vi "Read Absolute Max.vi"(8 "error in (no error)":errorcluster, 11 "PowerSupply in":refnum<class "PowerSupply.lvclass">) -> (0 "error out":errorcluster, 3 "PowerSupply out":refnum<class "PowerSupply.lvclass">)   [LabVIEW 2019, in "PowerSupply.lvlib" / "PowerSupply.lvclass"]
uses:
  PowerSupply.lvclass
  PowerSupply.lvclass/PowerSupply.ctl
  Accessors/Read/Read Configuration.vi
  Desktop/Built/Configuration.lvlibp/Configuration.lvclass
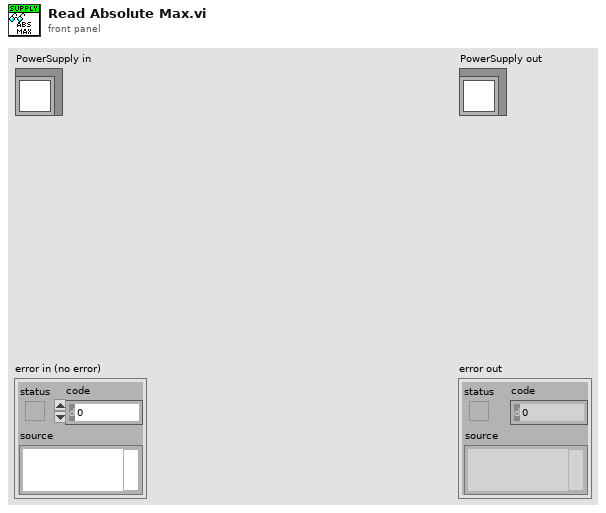
[diagram p1: front panel]
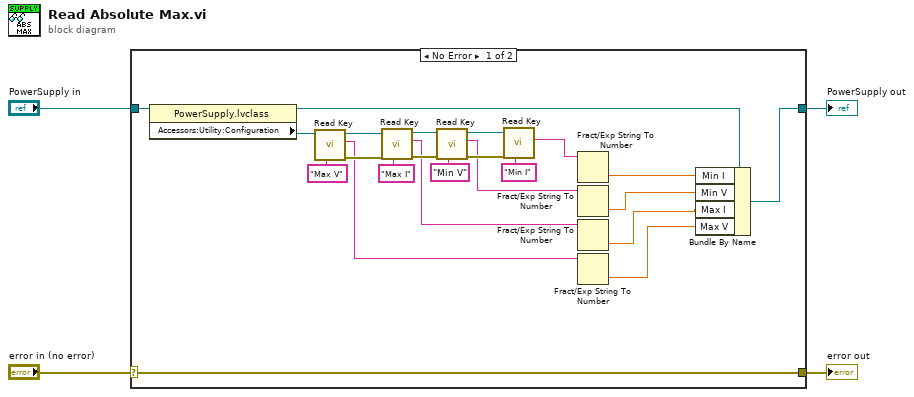
[diagram p0: block diagram]
diagram:
  n1 = case shown="No Error" "error in (no error)" {
    selector: "error in (no error)" -> [w26 w29]
    tunnel: [w26 w29] -> w3
    tunnel: [w13 w28] -> w1
    tunnel: "PowerSupply in" -> [w27 w28]
    frame No Error {
      n2 = property class="PowerSupply.lvclass"(reference=w27) -> (reference out=w25:refnum<class "PowerSupply.lvclass">, "Accessors:Utility:Configuration"=w24:refnum<class "Configuration.lvclass">)  [unwired: 1 in, 1 out]
      n3 = call "Read Key.vi"("Key Name"="Max V", "Configuration in"=w24) -> ("error out"=w22:errorcluster, "Key Value"=w8:string, "Configuration out"=w21:refnum<class "Configuration.lvclass">)  [unwired: 7 in]
      n4 = call "Read Key.vi"("Key Name"="Max I", "error in (no error)"=w22, "Configuration in"=w21) -> ("error out"=w17:errorcluster, "Key Value"=w9:string, "Configuration out"=w16:refnum<class "Configuration.lvclass">)  [unwired: 6 in]
      n5 = call "Read Key.vi"("Key Name"="Min V", "error in (no error)"=w17, "Configuration in"=w16) -> ("error out"=w18:errorcluster, "Key Value"=w10:string, "Configuration out"=w15:refnum<class "Configuration.lvclass">)  [unwired: 6 in]
      n6 = call "Read Key.vi"("Key Name"="Min I", "error in (no error)"=w18, "Configuration in"=w15) -> ("Key Value"=w11:string)  [unwired: 6 in, 2 out]
      n7 = Fract/Exp String To Number(string=w11) -> (number=w12:dbl)  [unwired: 3 in, 1 out]
      n8 = Fract/Exp String To Number(string=w10) -> (number=w7:dbl)  [unwired: 3 in, 1 out]
      n9 = Fract/Exp String To Number(string=w9) -> (number=w6:dbl)  [unwired: 3 in, 1 out]
      n10 = Fract/Exp String To Number(string=w8) -> (number=w5:dbl)  [unwired: 3 in, 1 out]
      n11 = Bundle By Name(cluster=w25, "Min I"=w12, "Min V"=w7, "Max I"=w6, "Max V"=w5) -> (w13:refnum<class "PowerSupply.lvclass">)
    }
    frame Error {
    }
  }
  "error out" <- w3
  "PowerSupply out" <- w1
